vi "HexConverter.vi"() -> ()   [LabVIEW 2009]
panel:
  out "Hex":u8 format="%.0x"
  in  "Decimal":u8
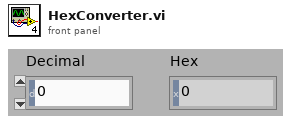
[diagram p1: front panel]
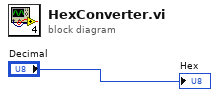
[diagram p0: block diagram]
diagram:
  "Hex" <- "Decimal"
